vi "ZPL Config Triggers.vi"(6 "Settle (1 mS)":u32=1, 7 "Trigger in Delay":dbl caption="TRIG:DELay" min=0.0 max=65.0 step=0.001, 8 "error":errorcluster, 9 "Trigger Out Mode":u16(ring) caption="OUTP:TTLT:MODE" items=["OFF", "TRIG", "FSTR"], 10 "Trigger in  Source":u16(ring) caption="TRIGger:SOURce" items=["EXT", "BUS"], 11 "VISA":refnum<visa-resource-name>) -> (0 "error out":errorcluster, 2 "final string":string, 3 "VISA out":refnum<visa-resource-name>)   [LabVIEW 2015]
doc: "This command selects the power supply input trigger source as follows:\n\" BUS (*TRG & TRIG) and Front Panel \n\" EXT Mainframe backplane Trigger IN PIN\n\nThis command sets the time delay between the detection of an event on the specified trigger source and the start of any corresponding trigger action on the power supply's output.\n\nThis command sets the operation of the Trigger Out signal to either OFF, Function Strobe or Trigger mode. Factory default is OFF.\n \n\nThis VI will wait for \"Settle\" milliseconds after setting the limit to allow the output to reach the new setting. If unwired, there will be no delay"
panel:
  # "Lambda ZPLUS \n Serial Port\n  DC Power Supplies"
  # "Configutate Input and Output Trigger"
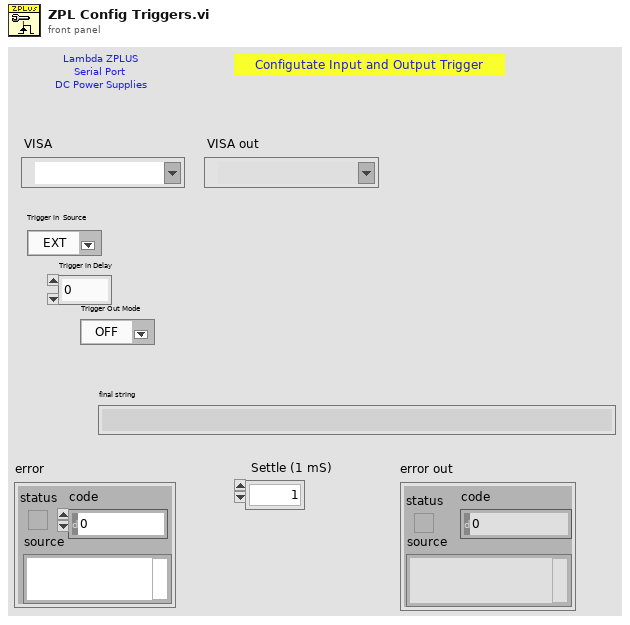
[diagram p1: front panel]
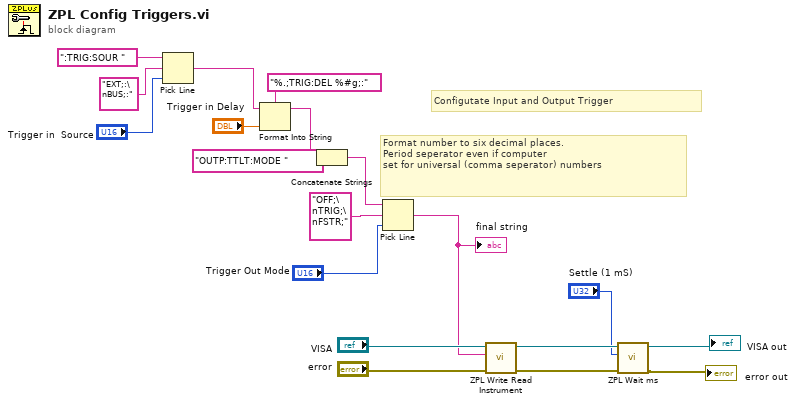
[diagram p0: block diagram]
diagram:
  # "Format number to six decimal places.\nPeriod seperator even if computer \nset for universal (comma seperator) numbers"
  # "Configutate Input and Output Trigger"
  n1 = Pick Line(string ("")=":TRIG:SOUR " ("format string"), multi-line string="EXT;:\nBUS;:" ("format string"), line index="Trigger in  Source") -> (output string=w8:string)
  n2 = Format Into String(format string="%.;TRIG:DEL %#g;:", initial string=w8, "Trigger in Delay") -> (resulting string=w4:string)  [unwired: 1 in, 1 out]
  n3 = Concatenate Strings(w4, "OUTP:TTLT:MODE " ("string")) -> (w3:string)
  n4 = Pick Line(string ("")=w3, multi-line string="OFF;\nTRIG;\nFSTR;" ("format string"), line index="Trigger Out Mode") -> (output string=w1:string)
  "final string" <- w1
  n5 = call "ZPL Write Read Instrument.vi"("error in"="error", "Write Command/Query SCPI"=w1, "VISA"="VISA") -> ("error out"=w16:errorcluster, "VISA  out"=w17:refnum<visa-resource-name>)  [unwired: 6 in, 1 out]
  n6 = call "ZPL Wait ms.vi"("error"=w16, "Delay (1 mS)"="Settle (1 mS)", "VISA"=w17) -> ("error out"=→"error out":errorcluster, "VISA out"=→"VISA out":refnum<visa-resource-name>)  [unwired: 7 in]
